vi "Add if New Else Append Single.vi"(9 "Cascaded Static Value":bool, 10 "New Element":T1, 11 "Style In":T1) -> (3 "Style Out":T1)   [LabVIEW 2019, in "LSS.lvlib"]
doc: "This VI finds takes a cluster of properties and adds new elements to it. Each new element is compared with the elements already in the cluster array to find out if it should be added as a new element or if it should override the element that is already there. \n\nThis essentially provides the cascading effect of more specific properties overriding more generic ones. Since the specifiers are pre-sorted in priority order, the most specific properties will always be the last ones to go through this sort.\n\nInputs:\n<b>Style In</b> - Cluster array of styles that have been found to apply to the current control.\n<b>New Element</b> - The new element found that should be added to the list.\n\nOutput:\n<b>Style Out</b> - Cluster array with new element properly added."
uses:
  LSS.lvlib
  Controls/Style.ctl
panel:
  out "Old":T2(array[cluster])
  out "New":T2(array[cluster])
  # "New and Old are troubleshooting outputs only."
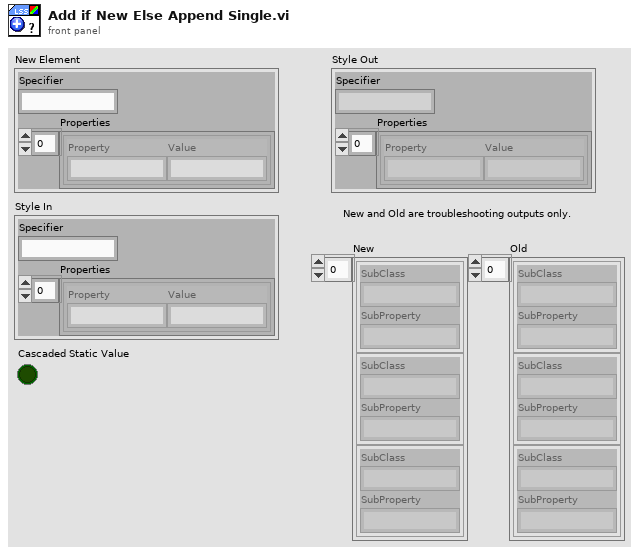
[diagram p1: front panel]
types:
  T1 = typedef "LSS.lvlib/Style.ctl" = cluster{"Specifier":string, "Properties":cluster{"Property":string, "Value":string}[]}
  T2 = cluster{"SubClass":string, "SubProperty":string}[]
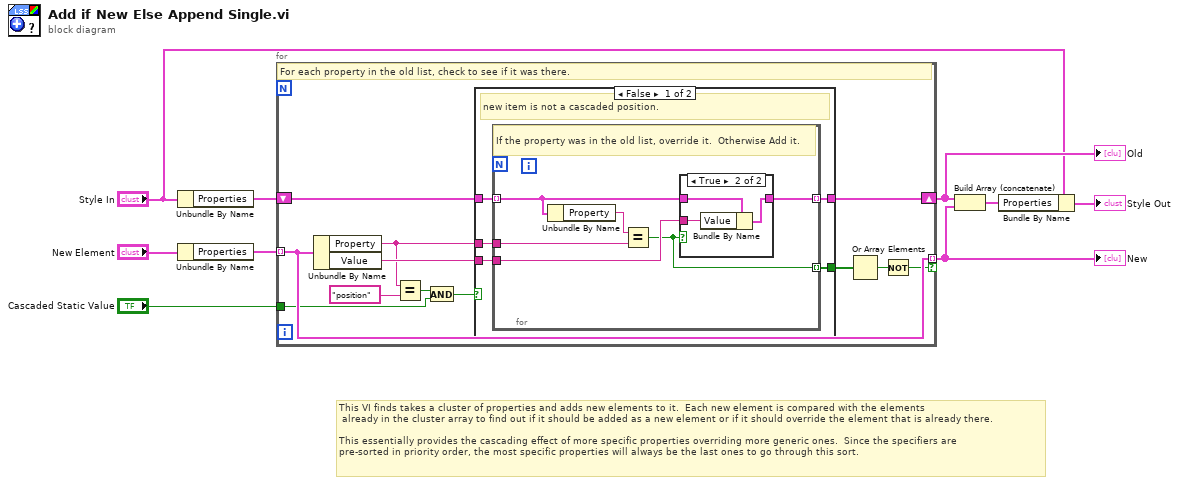
[diagram p0: block diagram]
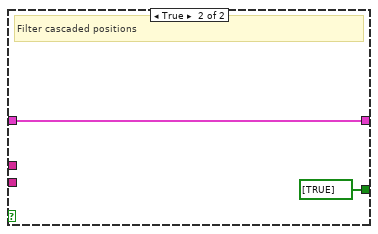
[diagram p3: hidden frame]
diagram:
  # "This VI finds takes a cluster of properties and adds new elements to it.  Each new element is compared with the elements\n already in the cluster array to find out if it should be added as a new element or if it should override the element that is already there.  \n\nThis essentially provides the cascading effect of more specific properties overriding more generic ones.  Since the specifiers are \npre-sorted in priority order, the most specific properties will always be the last ones to go through this sort."
  n1 = Unbundle By Name("Style In") -> ("Properties"=w7:cluster{"Property":string, "Value":string}[])
  n2 = Unbundle By Name("New Element") -> ("Properties"=w9:cluster{"Property":string, "Value":string}[])
  n3 = for {
    tunnel: w9 -> [w20] mode=indexing
    tunnel: [w20] -> w4 mode=indexing if=w19
    shift-right: [w17] -> w5
    shift-left: w7 -> [w21]
    tunnel: "Cascaded Static Value" -> [w13]
    # "For each property in the old list, check to see if it was there."
    n4 = Unbundle By Name(w20) -> ("Property"=w10:string, "Value"=w15:string)
    n5 = Equal?(x=w10, y="position") -> (x = y?=w14:bool)
    n6 = And(x=w14, y=w13) -> (x .and. y?=w11:bool)
    n7 = case shown="False" w11 {
      tunnel: w21 -> [w26 w38]
      tunnel: [w25 bool[] [TRUE]] -> w18
      tunnel: [w24 w38] -> w17
      tunnel: w15 -> [w23 _]
      tunnel: w10 -> [w22 _]
      frame False {
        # "new item is not a cascaded position."
        n8 = for {
          tunnel: w26 -> [w32] mode=indexing
          tunnel: [w27] -> w25 mode=indexing
          tunnel: [w31] -> w24 mode=indexing
          tunnel: w22 -> [w29]
          tunnel: w23 -> [w28]
          # "If the property was in the old list, override it.  Otherwise Add it."
          n9 = Unbundle By Name(w32) -> ("Property"=w30:string)
          n10 = Equal?(x=w30, y=w29) -> (x = y?=w27:bool)
          n11 = case shown="True" w27 {
            tunnel: w32 -> [w33 w36]
            tunnel: w28 -> [_ w35]
            tunnel: [w33 w34] -> w31
            frame False {
            }
            frame True {
              n12 = Bundle By Name(cluster=w36, "Value"=w35) -> (w34:cluster{"Property":string, "Value":string})
            }
          }
        }
      }
      frame True {
        # "Filter cascaded positions"
      }
    }
    n13 = Or Array Elements(Boolean array=w18) -> (logical OR=w16:bool)
    n14 = Not(x=w16) -> (.not. x?=w19:bool)
  }
  "Old" <- w5
  "New" <- w4
  n15 = Build Array (concatenate)(w5, w4) -> (w6:cluster{"Property":string, "Value":string}[])
  n16 = Bundle By Name(cluster="Style In", "Properties"=w6) -> (→"Style Out":T1)
